vi "Counter MC.vi"() -> (4 "b3":bool, 5 "b2":bool, 6 "b1":bool, 7 "bo":bool)   [LabVIEW 2012]
doc: "M. Corti 2004"
panel:
  in  "?":bool
  out "e":bool
  out "f":bool
  out "c":bool
  out "d":bool
  out "g":bool
  out "b":bool
  out "a":bool
  out "Clock":bool
  out "?":dbl
  out "3":bool
  out "2":bool
  out "1":bool
  out "0":bool
  out "?":cluster{i16, i16, i16, i16}(graph)
  # "Digital Output"
  # "4-Bit Binary Counter"
  # "0"
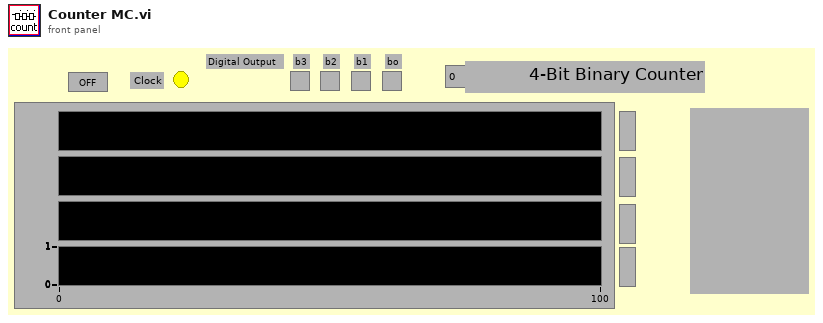
[diagram p1: front panel]
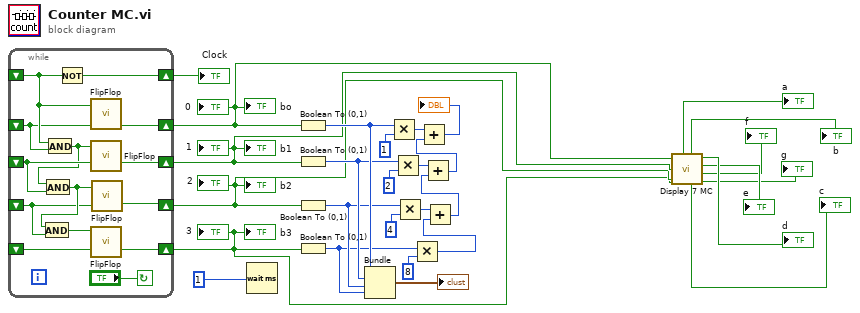
[diagram p0: block diagram]
diagram:
  n1 = while {
    shift-right: [w35] -> w11
    shift-left: _ -> [w31]
    shift-right: [w38] -> w10
    shift-left: _ -> [w43]
    shift-right: [w37] -> w9
    shift-left: _ -> [w41]
    shift-right: [w36] -> w8
    shift-left: _ -> [w39]
    shift-right: [w34] -> w12
    shift-left: _ -> [w32]
    stop <- "?" continue-if-true
    n2 = And(x=w32, y=w31) -> (x .and. y?=w33:bool)
    n3 = And(x=w33, y=w43) -> (x .and. y?=w42:bool)
    n4 = And(x=w42, y=w41) -> (x .and. y?=w40:bool)
    n5 = Not(x=w32) -> (.not. x?=w34:bool)
    n6 = call "FlipFlop.vi"("input"=w31, "clock"=w32) -> ("output"=w35:bool)
    n7 = call "FlipFlop.vi"("input"=w43, "clock"=w33) -> ("output"=w38:bool)
    n8 = call "FlipFlop.vi"("input"=w39, "clock"=w40) -> ("output"=w36:bool)
    n9 = call "FlipFlop.vi"("input"=w41, "clock"=w42) -> ("output"=w37:bool)
  }
  "bo" <- w11
  "b1" <- w10
  "b2" <- w9
  "b3" <- w8
  "0" <- w11
  "1" <- w10
  "2" <- w9
  "3" <- w8
  "Clock" <- w12
  n10 = Wait (ms)(milliseconds to wait=1) -> ()  [unwired: 1 out]
  n11 = Boolean To (0,1)(Boolean=w11) -> (0, 1=w26:i16)
  n12 = Boolean To (0,1)(Boolean=w10) -> (0, 1=w23:i16)
  n13 = Boolean To (0,1)(Boolean=w9) -> (0, 1=w20:i16)
  n14 = Boolean To (0,1)(Boolean=w8) -> (0, 1=w17:i16)
  n15 = Bundle(w26, w23, w20, w17) -> (→"?":cluster{i16, i16, i16, i16})  [unwired: 1 in]
  n16 = Multiply(x=w26, y=1) -> (x*y=w27:i32)
  n17 = Multiply(x=w23, y=2) -> (x*y=w24:i32)
  n18 = Multiply(x=w20, y=4) -> (x*y=w21:i32)
  n19 = Multiply(x=w17, y=8) -> (x*y=w18:i32)
  n20 = Add(x=w21, y=w18) -> (x+y=w14:i32)
  n21 = Add(x=w24, y=w14) -> (x+y=w15:i32)
  n22 = Add(x=w27, y=w15) -> (x+y=→"?":i32)
  n23 = call "Display 7 MC.vi"("b0"=w11, "b1"=w10, "b3"=w8, "b2"=w9) -> ("a"=→"a":bool, "b"=→"b":bool, "d"=→"d":bool, "e"=→"e":bool, "c"=→"c":bool, "f"=→"f":bool, "g"=→"g":bool)
